vi "Find Window Reference.vi"(8 "error in (no error)":errorcluster, 11 "VI Refnum":refnum<vi>) -> (0 "error out":errorcluster, 3 "Window Handle":refnum<k24>)   [LabVIEW 2015, in "Simple Progress Bar.lvlib"]
uses:
  Simple Progress Bar.lvlib
  User32.dll
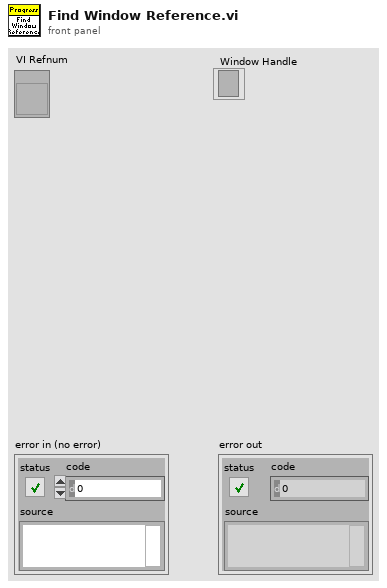
[diagram p1: front panel]
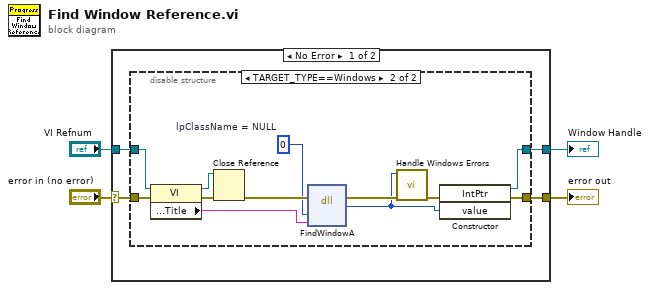
[diagram p0: block diagram]
diagram:
  n1 = case shown="No Error" "error in (no error)" {
    selector: "error in (no error)" -> [w7 w22]
    tunnel: "VI Refnum" -> [w8 _]
    tunnel: [w6 w22] -> w2
    tunnel: [w5 _] -> w1
    frame No Error {
      n2 = disable-structure shown="TARGET_TYPE==Windows" {
        disable-tunnel: w8 -> [_ w18]
        disable-tunnel: w7 -> [w9 w19]
        disable-tunnel: [w9 w11] -> w6
        disable-tunnel: [_ w10] -> w5
        frame condition #0 {
          # "#ToError"
        }
        frame condition #1 (active) {
          w16 = u32 0  # lpClassName = NULL
          n3 = property class="VI"(reference=w18, error in=w19) -> (reference out=w20:refnum<vi>, error out=w21:errorcluster, "Front Panel.Title"=w15:string)
          n4 = Close Reference(reference=w20, error in (no error)=w21) -> (error out=w17:errorcluster)
          n5 = dll-call lib="user32.dll" fn="FindWindowA"(error in=w17, "lpClassName"=w16, "lpWindowName"=w15) -> (error out=w14:errorcluster, "return type"=w12:i64)  [unwired: 4 in, 1 out]
          n6 = call "Handle Windows Errors.vi"("error in (no error)"=w14, "Handle"=w12) -> ("error out"=w13:errorcluster)  [unwired: 9 in]
          n7 = constructor class="IntPtr"(error in=w13, "value"=w12) -> (reference out=w10:refnum<k24>, error out=w11:errorcluster)  [unwired: 2 in, 2 out]
        }
      }
    }
    frame Error {
    }
  }
  "error out" <- w2
  "Window Handle" <- w1
